vi "3.4-How.vi"   [LabVIEW 2010]
uses:
  4-High Neurons/4.4-How Sensor Typedef.ctl
  4-High Neurons/4.0-Midbrain State.ctl
  <vilib>/rvi/interface/nirviReadWriteControl/nirviReadWriteControl.xnode
  2-Low Neurons/2-FPGA VI Typedef.ctl
  2-Low Neurons/2.4-How Sensor Typedef.ctl
  2-Low Neurons/2.1 Act Debug.ctl
  FPGA Bitfiles/DaveBrain_FPGATarget_1-Hindbrain_F0E489D8.lvbitx
  1-Hindbrain.vi
  <vilib>/rvi/interface/common/niFpgaNodeNameForErrorReporting.ctl
  <vilib>/rvi/errors/niLvFpgaWhatHappensToTopLevelVI.ctl
  3.0-Global.vi
  <vilib>/Utility/error.llb/Error Cluster From Error Code.vi
  <vilib>/rvi/errors/niLvFpgaAdjustHostInterfaceError.vi
  NiFpgaLv.dll
types:
  T1 = typedef "4.4-How Sensor Typedef.ctl" = cluster{"Motor Speed Integer":i32, "Drive Position Integer":i32, "Lidar Position Integer":i32, "Lidar Motor Position Integer":i32, "Steering Position Integer":i32, "Battery Voltage Fxp":dbl, "Drive Encoder Cable Check":bool, "Lidar Drive Encoder Cable Check":bool, "Steer Encoder Cable Check":bool, "Lidar Pos Encoder Cable Check":bool, "Mod Buttons & Blinky Cable Check":bool, "Lidar Data Cable Check":bool, "Drive Motor Cable Check":bool, "Vector Nav Cable Check":bool, "Lidar Drive Cable Check":bool, "Steer Drive Cable Check":bool, "Reverse?":bool, "2.1  Steering Control Voltage":dbl, "2.1 Drive Control Voltage":dbl, "2.1  Lidar Control Voltage":dbl, "2.5.7 A*B":dbl, "2.1  Steering PID Output":dbl, "2.1 Drive PID Output":dbl, "2.1  Lidar PID Output":dbl, "2.1.1 Drive Error":dbl, "2.1.1 Drive Error I":dbl, "2.1.1 Drive Error D":dbl, "2.1.2 Steering Error":dbl, "2.1.2 Steering Error I":dbl, "2.1.2 Steering Error D":dbl, "2.1.3 Lidar Error":dbl, "2.1.3 Lidar Error I":dbl, "2.1.3 Lidar Error D":dbl, "VectorNav Ack Query":bool, "VectorNav Read Byte":u8, "VectorNav Read Status":enum16{"Waiting", "Reading", "Done"}, "4.0-Midbrain State":T2}
  T2 = typedef "4.0-Midbrain State.ctl" = enum16{"Startup", "Waiting to Run", "Running-OlinOval", "Running-ChannelFollow", "Running-WallFollow", "Running-OpenTransit", "Running-Joystick Training", "Shutdown", "Restart", "New IP"}
  T3 = typedef "2.1 Act Debug.ctl" = cluster{"Drive":cluster{"2.1 Drive Control Voltage":fxp<+/-,20,5>, "2.1 Drive PID Output":fxp<+/-,20,5>, "2.1.1 Drive Error":fxp<+/-,18,1>, "2.1.1 Drive Error I":fxp<+/-,64,46>, "2.1.1 Drive Error D":fxp<+/-,18,1>, "Motor Speed Integer":fxp<+/-,10,8>, "Drive Position Integer":i32}, "Steering":cluster{"2.1  Steering Control Voltage":fxp<+/-,20,5>, "2.1  Steering PID Output":fxp<+/-,20,5>, "2.1.2 Steering Error":fxp<+/-,18,1>, "2.1.2 Steering Error I":fxp<+/-,64,46>, "2.1.2 Steering Error D":fxp<+/-,18,1>, "Steering V":fxp<+/-,10,8>, "Steering Position Integer":i32, "2.1  Steering V PID Output":fxp<+/-,20,5>, "2.1.2 Steering V Error":fxp<+/-,18,1>, "2.1.2 Steering V Error I":fxp<+/-,64,46>, "2.1.2 Steering V Error D":fxp<+/-,18,1>}, "Lidar":cluster{"2.1  Lidar Control Voltage":fxp<+/-,20,5>, "2.1  Lidar PID Output":fxp<+/-,20,5>, "2.1.3 Lidar Error":fxp<+/-,18,1>, "2.1.3 Lidar Error I":fxp<+/-,64,46>, "2.1.3 Lidar Error D":fxp<+/-,18,1>, "Lidar Position Integer":i32, "Lidar Motor Position Integer":i32}}
  T4 = typedef "2.4-How Sensor Typedef.ctl" = cluster{"Battery Voltage Fxp":fxp<+/-,16,5>, "Drive Encoder Cable Check":bool, "Lidar Drive Encoder Cable Check":bool, "Steer Encoder Cable Check":bool, "Lidar Pos Encoder Cable Check":bool, "Mod Buttons & Blinky Cable Check":bool, "Lidar Data Cable Check":bool, "Drive Motor Cable Check":bool, "Vector Nav Cable Check":bool, "Lidar Drive Cable Check":bool, "Steer Drive Cable Check":bool, "Reverse?":bool, "VectorNav Ack Query":bool, "VectorNav Read Byte":u8, "VectorNav Read Status":enum16{"Waiting", "Reading", "Done"}}
  T5 = typedef "niFpgaNodeNameForErrorReporting.ctl" = enum16{"Open FPGA VI Reference", "Read/Write Control", "Invoke Method: Abort", "Invoke Method: Acknowledge IRQ", "Invoke Method: Download", "Invoke Method: FIFO.Configure", "Invoke Method: FIFO.Read", "Invoke Method: FIFO.Start", "Invoke Method: FIFO.Stop", "Invoke Method: FIFO.Write", "Invoke Method: Reset", "Invoke Method: Run", "Invoke Method: Wait on IRQ", "Close FPGA VI Reference"}
  T6 = typedef "niLvFpgaWhatHappensToTopLevelVI.ctl" = enum16{"top level VI scripted behind XNode", "top level VI inlined behind XNode"}
  T7 = typedef "2-FPGA VI Typedef.ctl" = refnum<k20>
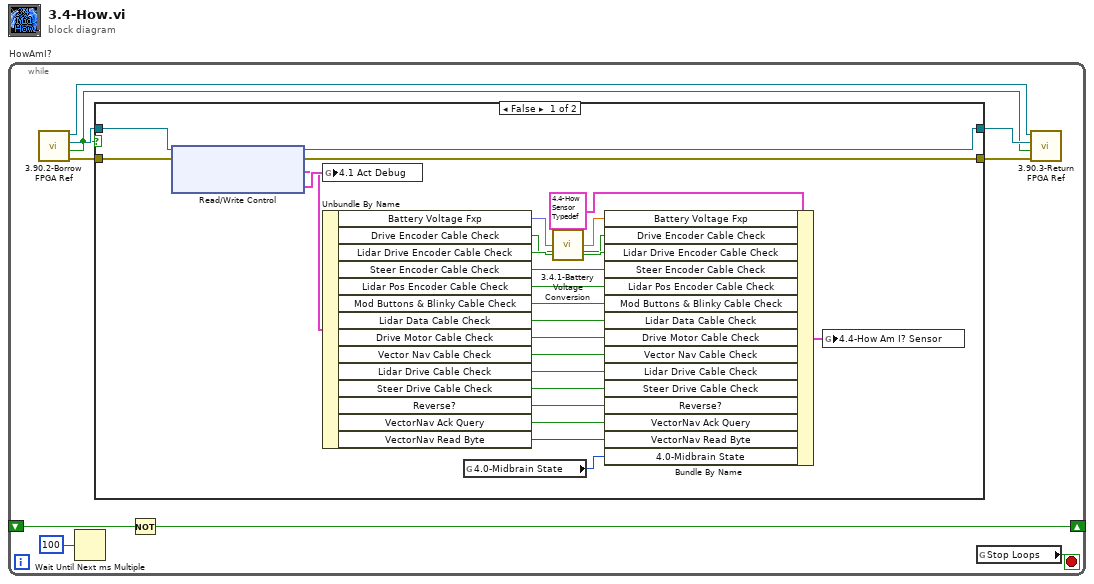
[diagram p0: block diagram]
diagram:
  n1 = while "HowAmI?" {
    shift-right: [w9] -> _
    shift-left: _ -> [w10]
    stop <- w1 stop-if-true
    n2 = call "3.90.2-Borrow FPGA Ref.vi"() -> ("error out"=w5:errorcluster, "Failed to Obtain Ref"=w2:bool, "element"=w8:T7, "FPGA Ref"=w7:refnum<queue>)  [unwired: 4 in]
    n3 = Wait Until Next ms Multiple(millisecond multiple=u32 100) -> ()  [unwired: 1 out]
    n4 = case shown="False" w2 {
      tunnel: w8 -> [w34 w117]
      tunnel: [w33 w117] -> w6
      tunnel: w5 -> [w32 w116]
      tunnel: [w31 w116] -> w4
      frame False {
        n5 = xnode "Read/Write Control"("FPGA VI Reference In"=w34, "error in"=w32) -> ("FPGA VI Reference Out"=w33:T7, "error out"=w31:errorcluster, "2.4 How Am I? Sensor"=w11:T4, "2.1 Act Debug"=w30:T3)
        n6 = global write "3.0-Global.vi" "4.1 Act Debug"(w30) -> ()
        n7 = Unbundle By Name(w11) -> ("Battery Voltage Fxp"=w25:fxp<+/-,16,5>, "Drive Encoder Cable Check"=w13:bool, "Lidar Drive Encoder Cable Check"=w14:bool, "Steer Encoder Cable Check"=w15:bool, "Lidar Pos Encoder Cable Check"=w16:bool, "Mod Buttons & Blinky Cable Check"=w17:bool, "Lidar Data Cable Check"=w18:bool, "Drive Motor Cable Check"=w19:bool, "Vector Nav Cable Check"=w20:bool, "Lidar Drive Cable Check"=w21:bool, "Steer Drive Cable Check"=w22:bool, "Reverse?"=w23:bool, "VectorNav Ack Query"=w29:bool, "VectorNav Read Byte"=w28:u8)
        n8 = global read "3.0-Global.vi" "4.0-Midbrain State"() -> (w27:T2)
        n9 = call "3.4.1-Battery Voltage Conversion.vi"("Input"=w25) -> ("Output"=w26:dbl)
        n10 = Bundle By Name(cluster=T1 {"Motor Speed Integer"=0, "Drive Position Integer"=0, "Lidar Position Integer"=0, "Lidar Motor Position Integer"=0, "Steering Position Integer"=0, "Battery Voltage Fxp"=0.0, "Drive Encoder Cable Check"=FALSE, "Lidar Drive Encoder Cable Check"=FALSE, "Steer Encoder Cable Check"=FALSE, "Lidar Pos Encoder Cable Check"=FALSE, "Mod Buttons & Blinky Cable Check"=FALSE, "Lidar Data Cable Check"=FALSE, "Drive Motor Cable Check"=FALSE, "Vector Nav Cable Check"=FALSE, "Lidar Drive Cable Check"=FALSE, "Steer Drive Cable Check"=FALSE, "Reverse?"=FALSE, "2.1  Steering Control Voltage"=0.0, "2.1 Drive Control Voltage"=0.0, "2.1  Lidar Control Voltage"=0.0, "2.5.7 A*B"=0.0, "2.1  Steering PID Output"=0.0, "2.1 Drive PID Output"=0.0, "2.1  Lidar PID Output"=0.0, "2.1.1 Drive Error"=0.0, "2.1.1 Drive Error I"=0.0, "2.1.1 Drive Error D"=0.0, "2.1.2 Steering Error"=0.0, "2.1.2 Steering Error I"=0.0, "2.1.2 Steering Error D"=0.0, "2.1.3 Lidar Error"=0.0, "2.1.3 Lidar Error I"=0.0, "2.1.3 Lidar Error D"=0.0, "VectorNav Ack Query"=FALSE, "VectorNav Read Byte"=0, "VectorNav Read Status"=enum."Waiting", "4.0-Midbrain State"=enum."Startup"} ("2.4 How Am I? Sensor"), "Battery Voltage Fxp"=w26, "Drive Encoder Cable Check"=w13, "Lidar Drive Encoder Cable Check"=w14, "Steer Encoder Cable Check"=w15, "Lidar Pos Encoder Cable Check"=w16, "Mod Buttons & Blinky Cable Check"=w17, "Lidar Data Cable Check"=w18, "Drive Motor Cable Check"=w19, "Vector Nav Cable Check"=w20, "Lidar Drive Cable Check"=w21, "Steer Drive Cable Check"=w22, "Reverse?"=w23, "VectorNav Ack Query"=w29, "VectorNav Read Byte"=w28, "4.0-Midbrain State"=w27) -> (w24:T1)
        n11 = global write "3.0-Global.vi" "4.4-How Am I? Sensor"(w24) -> ()
      }
      frame True {
      }
    }
    n12 = Not(x=w10) -> (.not. x?=w9:bool)
    n13 = global read "3.0-Global.vi" "Stop Loops"() -> (w1:bool)
    n14 = call "3.90.3-Return FPGA Ref.vi"("error in"=w4, "Failed to Obtain Ref"=w2, "element"=w6, "FPGA Ref"=w7) -> ()  [unwired: 1 out]
  }
